vi "lab_1_voloskov_kuznetsov.vi"(0 "Input 0":T3, 1 "Input 1":T3, 2 "Input 2":T3, 3 "Input 3":T3, 4 "Input 4":T3, 5 "Input":T3, 14 "Signal":T4) -> (6 "Output 0":T2, 7 "Output 4":T2, 8 "Output 1":T2, 9 "Output":T2, 10 "Output 2":T2, 12 "Output 3":T2, 15 "write_input":T1, 16 "write_output":T1)   [LabVIEW 2013]
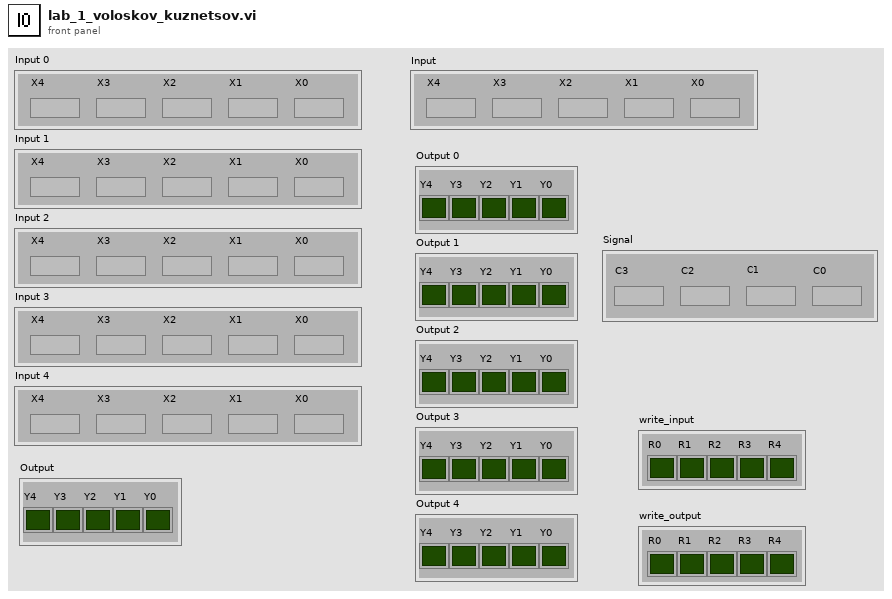
[diagram p1: front panel]
types:
  T1 = cluster{"R0":bool, "R1":bool, "R2":bool, "R3":bool, "R4":bool}
  T2 = cluster{"Y0":bool, "Y1":bool, "Y2":bool, "Y3":bool, "Y4":bool}
  T3 = cluster{"X0":bool, "X1":bool, "X2":bool, "X3":bool, "X4":bool}
  T4 = cluster{"C0":bool, "C1":bool, "C2":bool, "C3":bool}
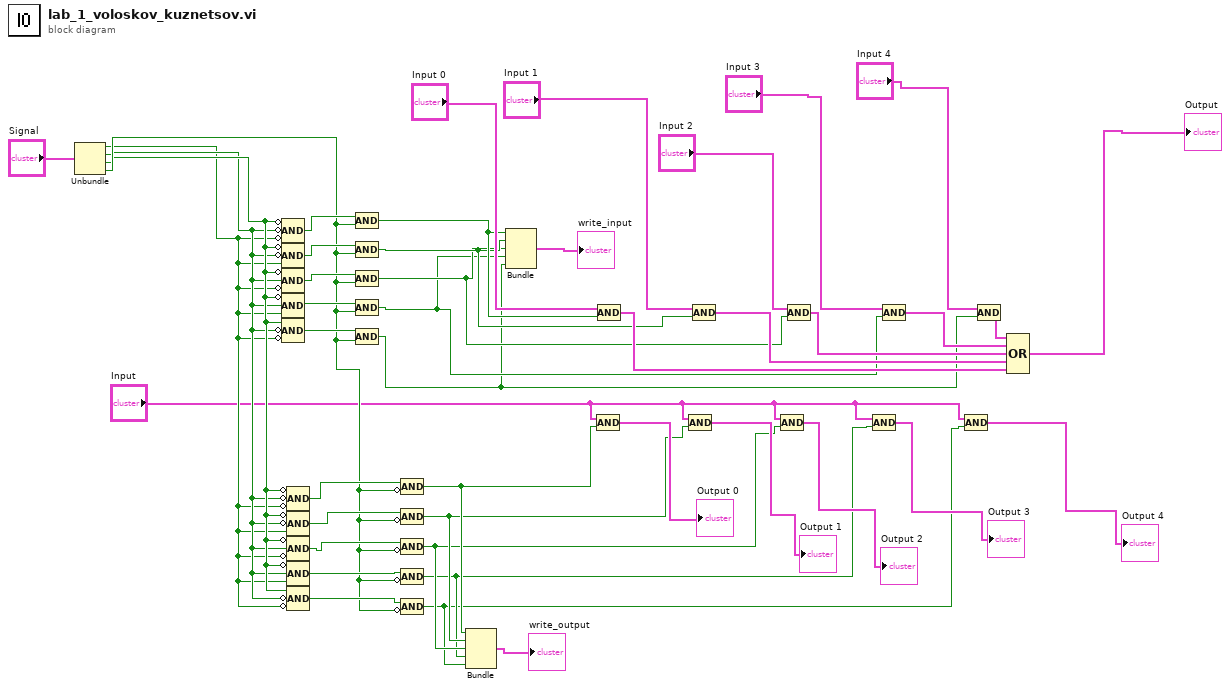
[diagram p0: block diagram]
diagram:
  n1 = Unbundle("Signal") -> ("C0"=w19:bool, "C1"=w20:bool, "C2"=w21:bool, "C3"=w22:bool)
  n2 = Compound Arithmetic op=AND(invert w21, invert w20, invert w19) -> (w35:bool)
  n3 = Compound Arithmetic op=AND(invert w21, invert w20, w19) -> (w36:bool)
  n4 = Compound Arithmetic op=AND(invert w21, w20, invert w19) -> (w37:bool)
  n5 = Compound Arithmetic op=AND(invert w21, w20, w19) -> (w38:bool)
  n6 = Compound Arithmetic op=AND(w21, invert w20, invert w19) -> (w39:bool)
  n7 = Compound Arithmetic op=AND(invert w21, invert w20, invert w19) -> (w34:bool)
  n8 = Compound Arithmetic op=AND(invert w21, invert w20, w19) -> (w33:bool)
  n9 = Compound Arithmetic op=AND(invert w21, w20, invert w19) -> (w32:bool)
  n10 = Compound Arithmetic op=AND(invert w21, w20, w19) -> (w31:bool)
  n11 = Compound Arithmetic op=AND(w21, invert w20, invert w19) -> (w30:bool)
  n12 = Compound Arithmetic op=AND(w35, w22) -> (w11:bool)
  n13 = Compound Arithmetic op=AND(w36, w22) -> (w10:bool)
  n14 = Compound Arithmetic op=AND(w37, w22) -> (w9:bool)
  n15 = Compound Arithmetic op=AND(w38, w22) -> (w8:bool)
  n16 = Compound Arithmetic op=AND(w39, w22) -> (w7:bool)
  n17 = Compound Arithmetic op=AND(w34, invert w22) -> (w5:bool)
  n18 = Compound Arithmetic op=AND(w33, invert w22) -> (w4:bool)
  n19 = Compound Arithmetic op=AND(w32, invert w22) -> (w3:bool)
  n20 = Compound Arithmetic op=AND(w31, invert w22) -> (w2:bool)
  n21 = Compound Arithmetic op=AND(w30, invert w22) -> (w1:bool)
  n22 = Bundle(w5, w4, w3, w2, w1) -> (→"write_output":cluster{bool, bool, bool, bool, bool})  [unwired: 1 in]
  n23 = Bundle(w11, w10, w9, w8, w7) -> (→"write_input":cluster{bool, bool, bool, bool, bool})  [unwired: 1 in]
  n24 = Compound Arithmetic op=AND("Input", w5) -> (→"Output 0":T3)
  n25 = Compound Arithmetic op=AND("Input 0", w11) -> (w40:T3)
  n26 = Compound Arithmetic op=AND("Input", w4) -> (→"Output 1":T3)
  n27 = Compound Arithmetic op=AND("Input 1", w10) -> (w41:T3)
  n28 = Compound Arithmetic op=AND("Input", w3) -> (→"Output 2":T3)
  n29 = Compound Arithmetic op=AND("Input 2", w9) -> (w42:T3)
  n30 = Compound Arithmetic op=AND("Input", w2) -> (→"Output 3":T3)
  n31 = Compound Arithmetic op=AND("Input 3", w8) -> (w43:T3)
  n32 = Compound Arithmetic op=AND("Input", w1) -> (→"Output 4":T3)
  n33 = Compound Arithmetic op=AND("Input 4", w7) -> (w44:T3)
  n34 = Compound Arithmetic op=OR(w44, w43, w42, w41, w40) -> (→"Output":T3)
